vi "GUI_HPDMAP2.vi"() -> ()   [LabVIEW 2020]
uses:
  Shared/GUI_Template/GUI_master/tcp_new_data_event.ctl
  Shared/GUI_Template/GUI_master/tcp new data cluster.ctl
panel:
  in  "HPDCCD2":bool
  in  "HPDCCD":bool
  in  "HeatHPDCCD":bool
  in  "HPDHolywedge":bool
  in  "HeatM3":bool
  in  "M3HPD":bool
  in  "Position.Channel 4::2":T1(ring) caption="Fiber"
  in  "Position.Channel 7::2":T1(ring) caption="Little Rick"
  in  "Position.Channel 6::2":T1(ring) caption="Big Franco"
  in  "Position.Channel 5::2":T1(ring) caption="Frog Foil"
  in  "Position.Channel 1::2":T1(ring) caption="Mipper"
  in  "pos.Channel11::3":enum16{"1", "2", "3", "4", "5", "6"}(ring) caption="HolyWedgecam"
  in  "pos.Channel3::3":enum16{"1", "2", "3", "4", "5", "6"}(ring) caption="HPD-Frog"
  in  "pos.Channel2::3":enum16{"1", "2", "3", "4", "5", "6"}(ring) caption="M3-Near"
  in  "pos.Channel9::3":enum16{"1", "2", "3", "4", "5", "6"}(ring) caption="HeatM3Near"
  in  "pos.Channel10::3":enum16{"1", "2", "3", "4", "5", "6"}(ring) caption="HPDCCD-FW3"
  in  "pos.Channel1::3":enum16{"1", "2", "3", "4", "5", "6"}(ring) caption="HPDCCD-HDR"
  in  "pos.Channel0::3":enum16{"1", "2", "3", "4", "5", "6"}(ring) caption="HPDCCD-Course"
  in  "pos.Channel12::3":enum16{"1", "2", "3", "4", "5", "6"}(ring) caption="HPD-HASO2"
  in  "pos.Channel7::3":enum16{"1", "2", "3", "4", "5", "6"}(ring) caption="HPD-HASO"
  in  "pos.Channel5::3":enum16{"1", "2", "3", "4", "5", "6"}(ring) caption="HPDCCD-2"
  in  "pos.Channel8::3":enum16{"1", "2", "3", "4", "5", "6"}(ring) caption="Heat-CCD"
  in  "position::5":dbl caption="HPD Far Stage Position" min=0.0 max=600.0 format="%#_6p"
  in  "GUIdevice 5":string="STAGE-HPD-Far"
  out "ypos":i32
  out "xpos":i32
  out "appargs 2":string[](array[string])
  in  "GUIdevice 2":string="1Wire"
  in  "save::2":bool caption="Blank Button"
  in  "trigger::2":bool caption="Blank Button"
  in  "GUIdevice 4":string="EM-HPD-1"
  in  "GUIdevice 3":string="FW-BELLA-General"
  in  "position::1":dbl caption="HPD Telescope Position" min=0.0 max=600.0 format="%#_6p"
  in  "GUIdevice 1":string="STAGE-HPD-Tel"
  in  "stop":bool
  out "error IO 2":errorcluster
  out "tcp data event":T2
  # "HPD Area MAP"
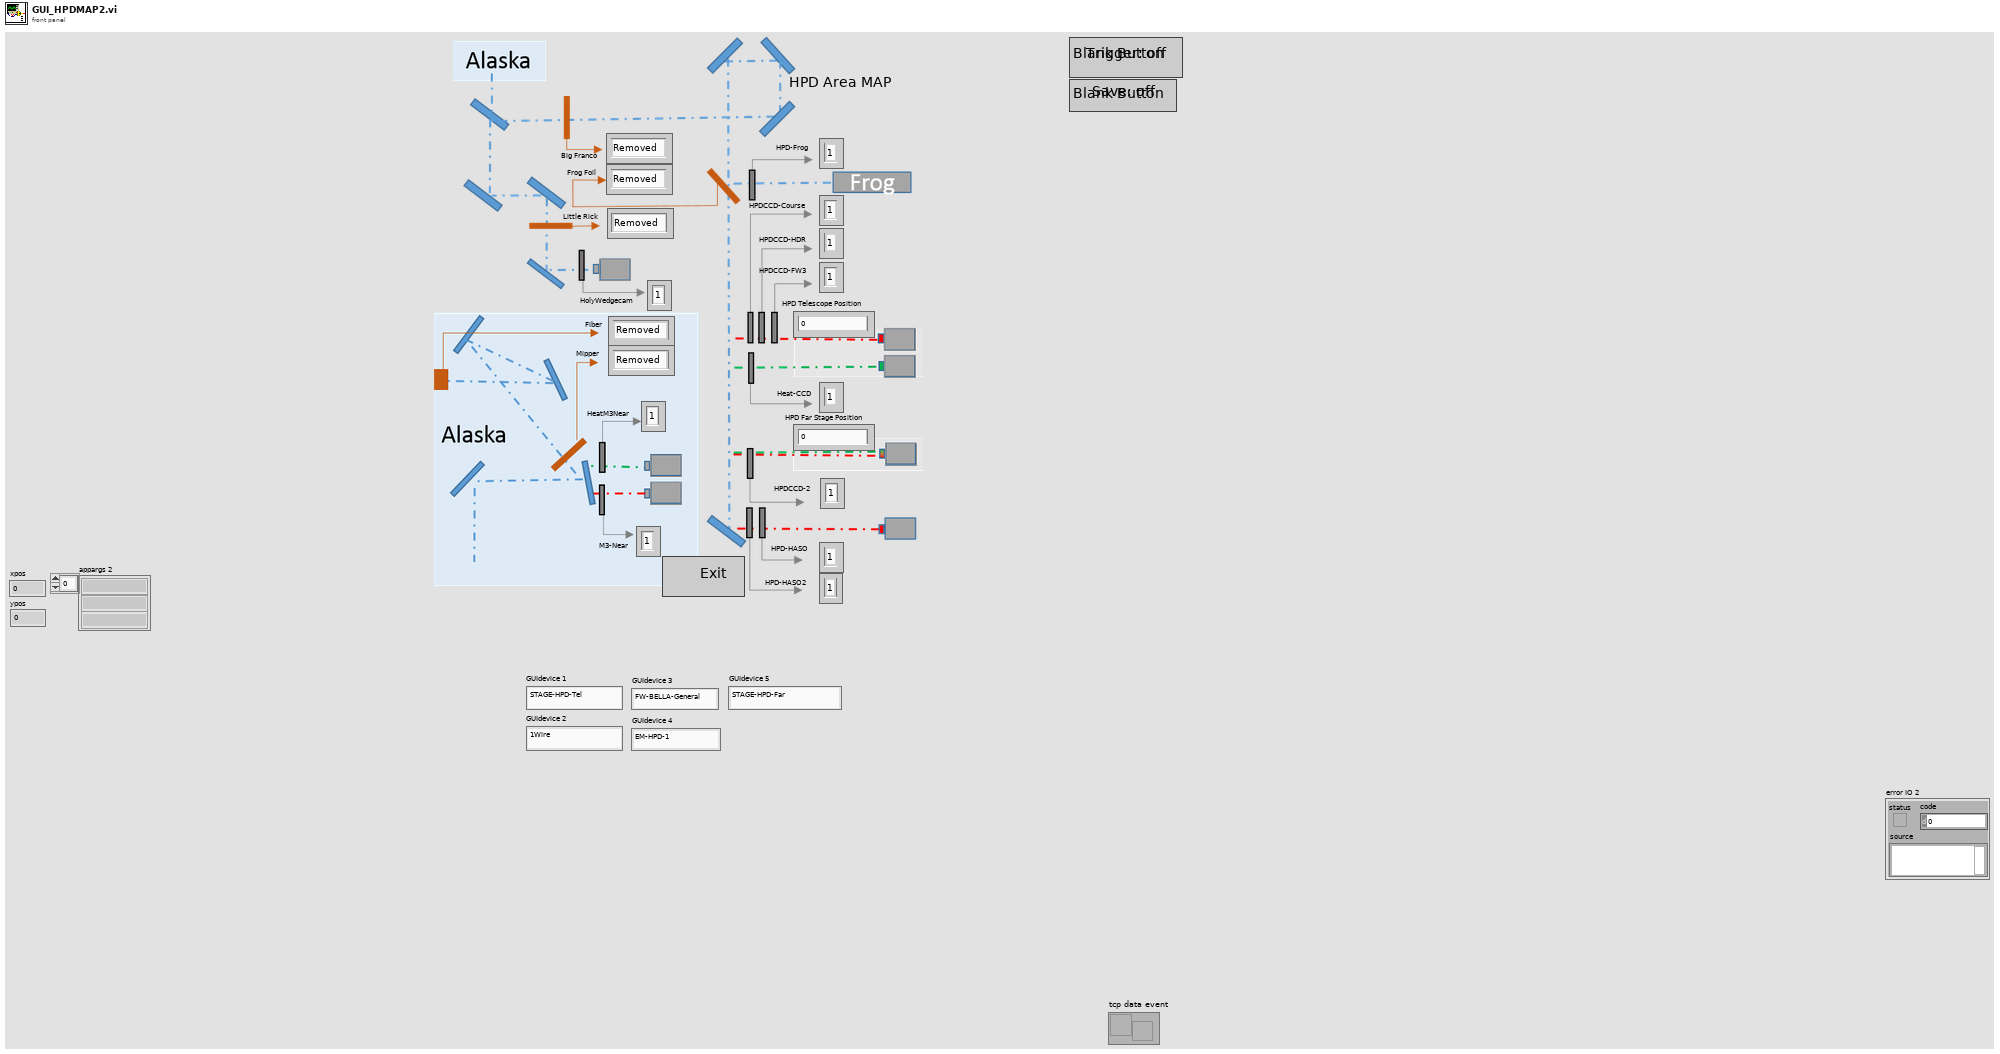
[diagram p1: front panel]
types:
  T1 = enum16{"Removed", "Inserted", "Unknown", "Moving"}
  T2 = typedef "tcp_new_data_event.ctl" = refnum<user-event>
  T3 = typedef "Image Type" = u32
  T4 = typedef "tcp new data cluster.ctl" = cluster{"EventEnum":enum16{"new data", "connection status update"}, "Device name":string}
  T5 = typedef "IMAQ Image.ctl" = refnum<image>
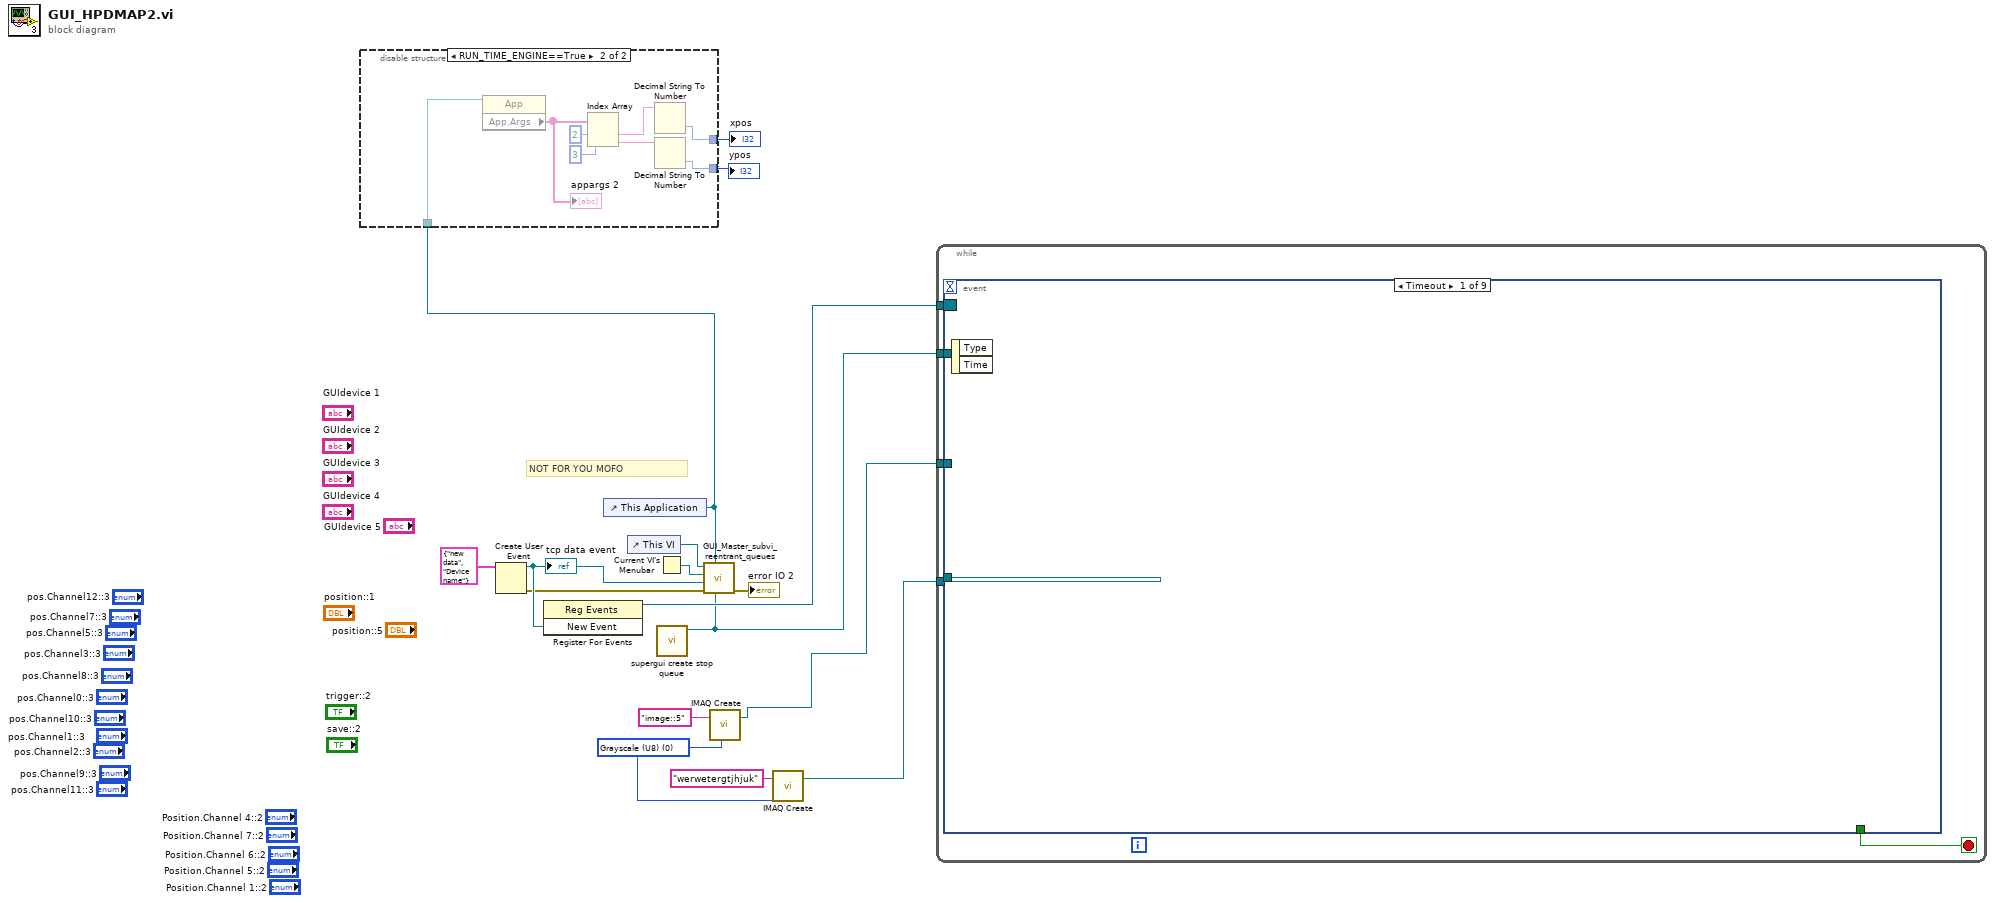
[diagram p0: block diagram]
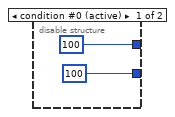
[diagram p2: hidden frame]
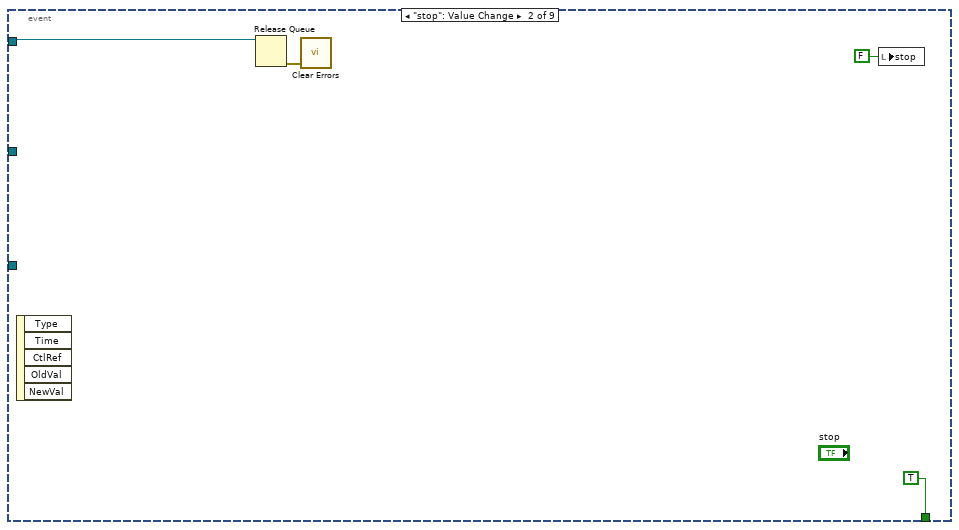
[diagram p3: hidden frame]
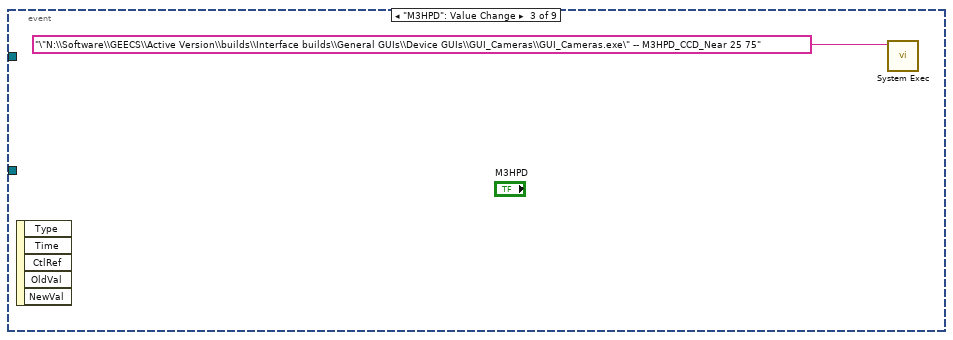
[diagram p4: hidden frame]
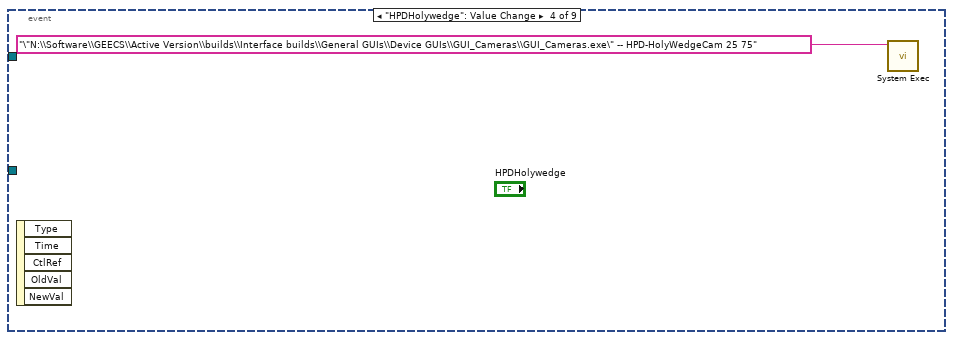
[diagram p5: hidden frame]
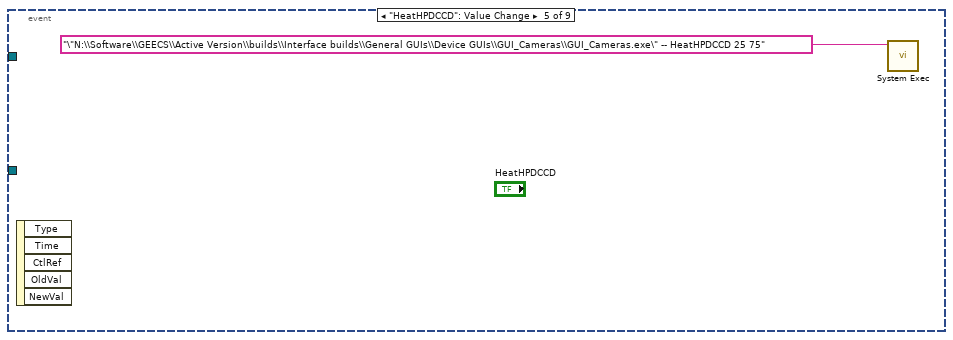
[diagram p6: hidden frame]
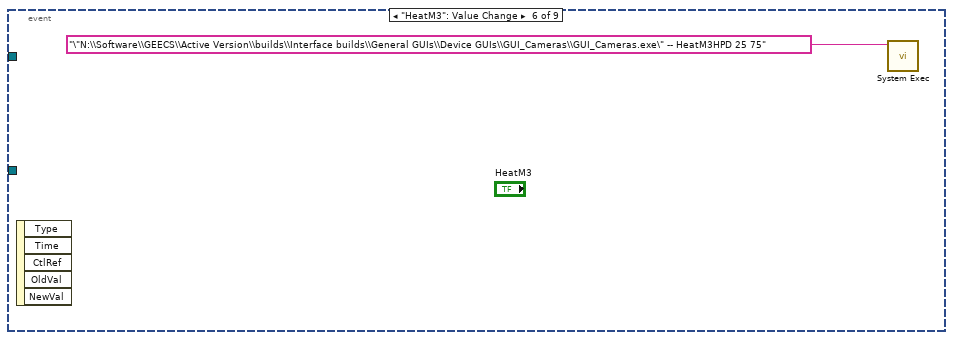
[diagram p7: hidden frame]
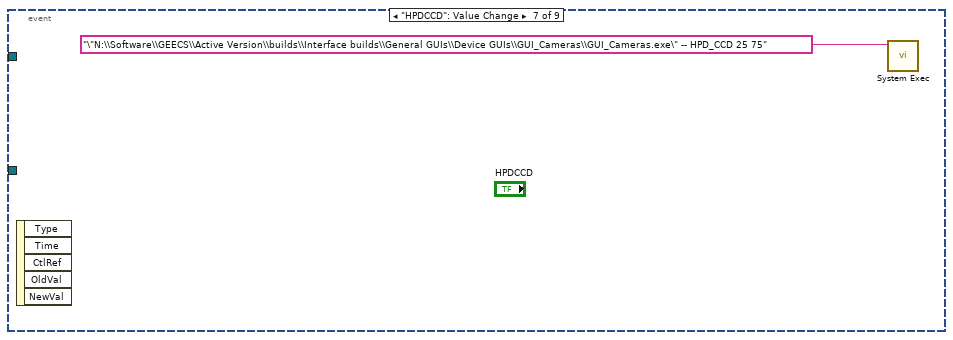
[diagram p8: hidden frame]
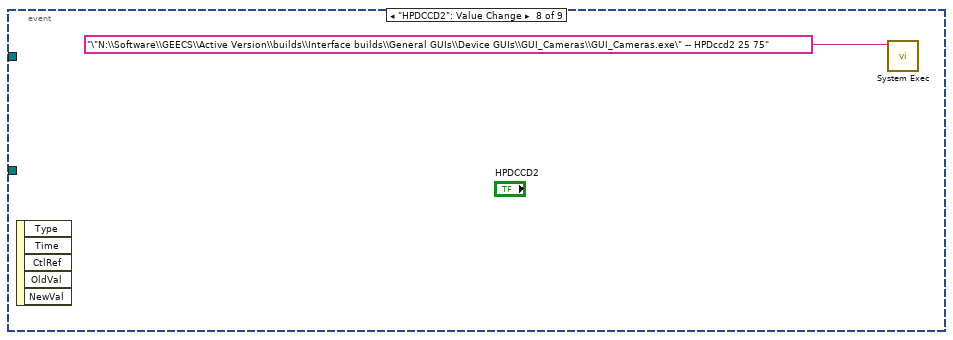
[diagram p9: hidden frame]
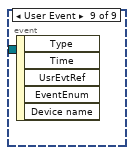
[diagram p10: hidden frame]
diagram:
  w4 = T3 0 items=["Grayscale (U8)", "Grayscale (I16)", "Grayscale (SGL)", "Complex (CSG)", "RGB (U32)", "HSL (U32)", "RGB (U64)", "Grayscale (U16)"] ("Image Type")
  # "NOT FOR YOU MOFO"
  n1 = Create User Event(user event datatype=T4 {"EventEnum"=enum."new data", "Device name"="Device name"} ("New Event")) -> (user event=w16:refnum<user-event>, error out=w15:errorcluster)  [unwired: 1 in]
  "tcp data event" <- w16
  n2 = register-events(w16) -> (reference out=w10:refnum<event-registration>)  [unwired: 2 in, 1 out]
  n3 = control-ref of="This Application"() -> (w9:refnum<vi>)
  n4 = disable-structure shown="RUN_TIME_ENGINE==True" {
    disable-tunnel: [100 ("number") w21] -> w8
    disable-tunnel: [100 ("number") w20] -> w7
    disable-tunnel: w9 -> [_ w19]
    frame condition #0 (active) {
    }
    frame condition #1 {
      n5 = property class="App"(reference=w19) -> ("App.Args"=w26:string[])  [unwired: 1 in, 2 out]
      "appargs 2" <- w26
      n6 = Index Array(array=w26, index #1=2 ("index"), index #2=3 ("index")) -> (element #1=w25:string, element #2=w24:string)
      n7 = Decimal String To Number(string=w25) -> (number=w21:i32)  [unwired: 2 in, 1 out]
      n8 = Decimal String To Number(string=w24) -> (number=w20:i32)  [unwired: 2 in, 1 out]
    }
  }
  "xpos" <- w8
  "ypos" <- w7
  n9 = control-ref of="This VI"() -> (w12:refnum<vi>)
  n10 = Current VI's Menubar() -> (w13:refnum<k9>)
  n11 = call "supergui create stop queue.vi"() -> ("STOP Queue out"=w1:refnum<queue>)  [unwired: 11 in]
  n12 = call "GUI_Master_subvi_reentrant_queues.vi"("STOP Queue in"=w1, "This Application"=w9, "error in (no error)"=w15, "tcp data event"=w16, "Caller menu reference"=w13, "Caller VI ref"=w12) -> ("error out"=→"error IO 2":errorcluster)  [unwired: 5 in]
  n13 = call "IMAQ Create"("Image Name"="image::5", "Image Type"=w4) -> ("New Image"=w2:T5)  [unwired: 3 in, 1 out]
  n14 = call "IMAQ Create"("Image Name"="werwetergtjhjuk", "Image Type"=w4) -> ("New Image"=w3:T5)  [unwired: 3 in, 1 out]
  n15 = while {
    tunnel: w10 -> [w30]
    tunnel: w3 -> [w29]
    tunnel: w2 -> [w28]
    tunnel: w1 -> [w27]
    stop <- w31 stop-if-true
    n16 = event shown="[0] Timeout" {
      selector: w30 -> [_ _ _ _ _ _ _ _ _]
      dyn-events: _ -> [_ _ _ _ _ _ _ _ _]
      timeout: _ -> [_ _ _ _ _ _ _ _ _]
      tunnel: [_ TRUE _ _ _ _ _ _ _] -> w31
      tunnel: w29 -> [_ _ _ _ _ _ _ _ _]
      tunnel: w28 -> [_ _ _ _ _ _ _ _ _]
      tunnel: w27 -> [_ w33 _ _ _ _ _ _ _]
      event Timeout {
        n17 = event-data() -> ()  [unwired: 1 in, 2 out]
      }
      event "stop": Value Change {
        n18 = event-data() -> ()  [unwired: 1 in, 5 out]
        n19 = Release Queue(queue=w33) -> (error out=w32:errorcluster)  [unwired: 2 in, 2 out]
        n20 = call <vilib>:"Clear Errors.vi"("error in (no error)"=w32) -> ()  [unwired: 5 in, 2 out]
        n21 = local write "stop"(FALSE ("stop")) -> ()
      }
      event "M3HPD": Value Change {
        n22 = event-data() -> ()  [unwired: 1 in, 5 out]
        n23 = call <vilib>:"System Exec.vi"("command line"="\"N:\\Software\\GEECS\\Active Version\\builds\\Interface builds\\General GUIs\\Device GUIs\\GUI_Cameras\\GUI_Cameras.exe\" -- M3HPD_CCD_Near 25 75") -> ()  [unwired: 7 in, 4 out]
      }
      event "HPDHolywedge": Value Change {
        n24 = event-data() -> ()  [unwired: 1 in, 5 out]
        n25 = call <vilib>:"System Exec.vi"("command line"="\"N:\\Software\\GEECS\\Active Version\\builds\\Interface builds\\General GUIs\\Device GUIs\\GUI_Cameras\\GUI_Cameras.exe\" -- HPD-HolyWedgeCam 25 75") -> ()  [unwired: 7 in, 4 out]
      }
      event "HeatHPDCCD": Value Change {
        n26 = event-data() -> ()  [unwired: 1 in, 5 out]
        n27 = call <vilib>:"System Exec.vi"("command line"="\"N:\\Software\\GEECS\\Active Version\\builds\\Interface builds\\General GUIs\\Device GUIs\\GUI_Cameras\\GUI_Cameras.exe\" -- HeatHPDCCD 25 75") -> ()  [unwired: 7 in, 4 out]
      }
      event "HeatM3": Value Change {
        n28 = event-data() -> ()  [unwired: 1 in, 5 out]
        n29 = call <vilib>:"System Exec.vi"("command line"="\"N:\\Software\\GEECS\\Active Version\\builds\\Interface builds\\General GUIs\\Device GUIs\\GUI_Cameras\\GUI_Cameras.exe\" -- HeatM3HPD 25 75") -> ()  [unwired: 7 in, 4 out]
      }
      event "HPDCCD": Value Change {
        n30 = event-data() -> ()  [unwired: 1 in, 5 out]
        n31 = call <vilib>:"System Exec.vi"("command line"="\"N:\\Software\\GEECS\\Active Version\\builds\\Interface builds\\General GUIs\\Device GUIs\\GUI_Cameras\\GUI_Cameras.exe\" -- HPD_CCD 25 75") -> ()  [unwired: 7 in, 4 out]
      }
      event "HPDCCD2": Value Change {
        n32 = event-data() -> ()  [unwired: 1 in, 5 out]
        n33 = call <vilib>:"System Exec.vi"("command line"="\"N:\\Software\\GEECS\\Active Version\\builds\\Interface builds\\General GUIs\\Device GUIs\\GUI_Cameras\\GUI_Cameras.exe\" -- HPDccd2 25 75") -> ()  [unwired: 7 in, 4 out]
      }
      event User Event {
        n34 = event-data() -> ()  [unwired: 1 in, 5 out]
      }
    }
  }
